vi "CAL-Test Against Exemplar.vi"(0 "Test file":path, 5 "Exemplar file":path, 7 "Tolerance (dB)":dbl, 11 "error in":errorcluster) -> (15 "error out":errorcluster)   [LabVIEW 2015]
uses:
  <vilib>/Analysis/5stat.llb/RMS (DBL).vi
  Utility VIs/Comparison VIs/Approx Equal (Scalar).vi
  <vilib>/Analysis/NI_AALPro.lvlib
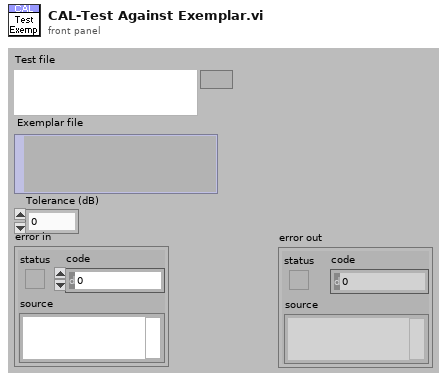
[diagram p1: front panel]
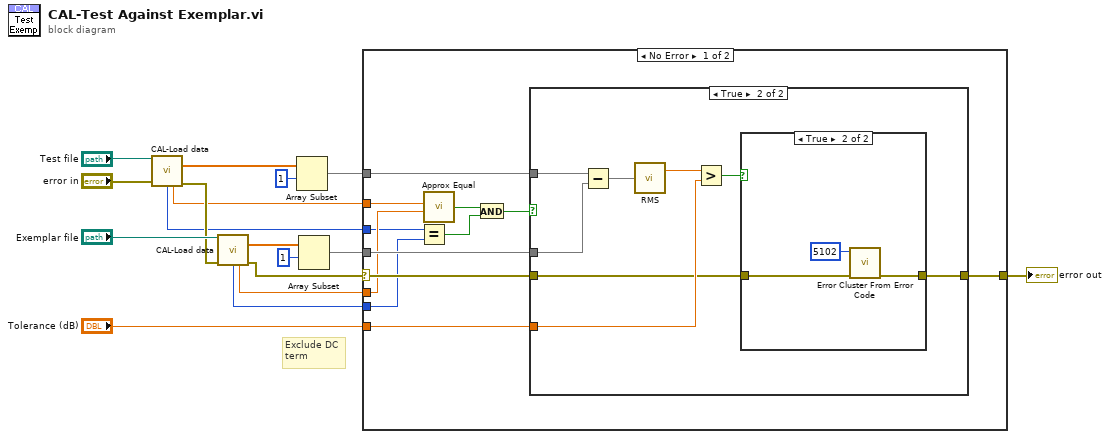
[diagram p0: block diagram]
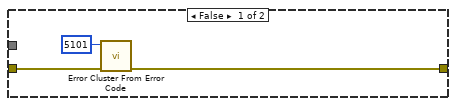
[diagram p2: hidden frame]
diagram:
  # "Exclude DC\nterm"
  n1 = call "CAL-Load data.vi"("user path"="Test file", "error in (no error)"="error in") -> ("Mag"=w8:dbl[], "npts"=w9:i32, "Fs (Hz)"=w12:dbl, "error out"=w14:errorcluster)  [unwired: 6 in, 4 out]
  n2 = call "CAL-Load data.vi"("user path"="Exemplar file", "error in (no error)"=w14) -> ("Mag"=w7:dbl[], "npts"=w10:i32, "Fs (Hz)"=w11:dbl, "error out"=w13:errorcluster)  [unwired: 6 in, 4 out]
  n3 = Array Subset(array=w8, index=1) -> (w4:dbl[])  [unwired: 1 in]
  n4 = Array Subset(array=w7, index=1) -> (w2:dbl[])  [unwired: 1 in]
  n5 = case shown="No Error" w13 {
    selector: w13 -> [w29 w45]
    tunnel: w12 -> [w27 _]
    tunnel: w11 -> [w26 _]
    tunnel: w10 -> [w25 _]
    tunnel: w9 -> [w24 _]
    tunnel: w4 -> [w18 _]
    tunnel: w2 -> [w28 _]
    tunnel: "Tolerance (dB)" -> [w20 _]
    tunnel: [w19 w45] -> w5
    frame No Error {
      n6 = Equal?(x=w24, y=w25) -> (x = y?=w22:bool)
      n7 = call-poly "Approx Equal.vi"("Y"=w26, "X"=w27) -> ("X approx Y?"=w23:bool)  [unwired: 4 in]
      n8 = And(x=w23, y=w22) -> (x .and. y?=w21:bool)
      n9 = case shown="True" w21 {
        tunnel: w18 -> [_ w40]
        tunnel: w28 -> [_ w39]
        tunnel: w29 -> [w32 w34]
        tunnel: w20 -> [_ w36]
        tunnel: [w30 w33] -> w19
        frame False {
          n10 = call <vilib>:"Error Cluster From Error Code.vi"("error in (no error)"=w32, "error code (0)"=5101) -> ("error out"=w30:errorcluster)  [unwired: 7 in]
        }
        frame True {
          n11 = Subtract(x=w40, y=w39) -> (x-y=w38:dbl[])
          n12 = call-poly <vilib>:"RMS.vi"("X"=w38) -> ("rms value"=w37:dbl)  [unwired: 1 out]
          n13 = Greater?(x=w37, y=w36) -> (0:w35:bool)
          n14 = case shown="True" w35 {
            tunnel: w34 -> [w41 w44]
            tunnel: [w41 w43] -> w33
            frame False {
            }
            frame True {
              n15 = call <vilib>:"Error Cluster From Error Code.vi"("error in (no error)"=w44, "error code (0)"=5102) -> ("error out"=w43:errorcluster)  [unwired: 7 in]
            }
          }
        }
      }
    }
    frame Error {
    }
  }
  "error out" <- w5
